vi "SP Matrix To Array - CM.vi"(1 "Complex Matrix":T1) -> (0 "Complex 2D Array":cdb[][](array[numeric]))   [LabVIEW 2011]
doc: "Converts a matrix of elements to an array of elements of the same data type. The data type you wire to the <B>Real Matrix</B> input determines the polymorphic instance to use."
uses:
  TypeDefs/SP Complex Matrix.ctl
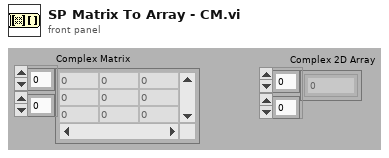
[diagram p1: front panel]
types:
  T1 = typedef "SP Complex Matrix.ctl" = cdb[][]
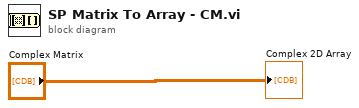
[diagram p0: block diagram]
diagram:
  "Complex 2D Array" <- "Complex Matrix"
